vi "_sendCommand.vi"(8 "FBLR":dbl[](array[numeric]), 11 "error in (no error)":errorcluster) -> (3 "error out":errorcluster)   [LabVIEW 2021, in "System.lvclass"]
uses:
  System.lvclass
  <vilib>/myRIO/Instrument Drivers/Onboard IO/AO/typedefs/AO Reference.ctl
  <vilib>/myRIO/Common/Instrument Driver Framework/Utilities/typedefs/myRIO Generic Hardware Reference.ctl
  <vilib>/myRIO/Common/Instrument Driver Framework/Utilities/typedefs/Hardware Version Enum.ctl
  <vilib>/myRIO/Common/Instrument Driver Framework/Utilities/typedefs/myRIO v1.0 Reference.ctl
  <vilib>/myRIO/Common/Instrument Driver Framework/Utilities/typedefs/Generic FPGA Reference.ctl
  <vilib>/myRIO/Common/Instrument Driver Framework/myRIO v1.0/AO/typedefs/AO Channels List.ctl
  <vilib>/myRIO/Common/Instrument Driver Framework/myRIO v1.0/AO/typedefs/AO Channels Enum.ctl
  <vilib>/myRIO/Common/Instrument Driver Framework/Utilities/typedefs/Analog Scaling Constants List.ctl
  <vilib>/myRIO/Common/Instrument Driver Framework/Utilities/typedefs/Analog Scaling Constants.ctl
  <vilib>/userDefined/High Color/nirio_resource_hc.ctl
  <vilib>/myRIO/Common/Instrument Driver Framework/Utilities/vis/Is FPGA Ref Available.vi
  <vilib>/myRIO/Common/Instrument Driver Framework/myRIO v1.0/AO/vis/myRIO v1.1 Open AO.vi
  <vilib>/myRIO/Instrument Drivers/Onboard IO/AO/vis/Write.vi
  <vilib>/myRIO/Common/Instrument Driver Framework/Utilities/vis/Validate Channels.vi
  <vilib>/myRIO/Common/Instrument Driver Framework/myRIO v1.0/AO/vis/myRIO v1.0 Reserve AO.vi
  <vilib>/myRIO/Common/Instrument Driver Framework/myRIO v1.0/AO/vis/myRIO v1.0 Build MUX Configuration AO.vi
  <vilib>/myRIO/Common/Instrument Driver Framework/myRIO v1.0/Resource Manager/vis/myRIO v1.0 Reserve Channel List.vi
  <vilib>/myRIO/Common/Instrument Driver Framework/myRIO v1.0/Resource Manager/vis/myRIO v1.0 Reserve Channel.vi
  <vilib>/myRIO/Common/Instrument Driver Framework/myRIO v1.0/Resource Manager/vis/myRIO v1.0 Unreserve Channel.vi
  <vilib>/myRIO/Common/Instrument Driver Framework/myRIO v1.0/Resource Manager/vis/myRIO v1.0 Build Mutex Name.vi
  <vilib>/Utility/VariantDataType/GetNumericInfo.vi
  <vilib>/Utility/error.llb/Error Cluster From Error Code.vi
  <vilib>/myRIO/Common/Instrument Driver Framework/myRIO v1.0/myRIO v1.1 Open.vi
  <vilib>/myRIO/Common/Instrument Driver Framework/myRIO v1.0/AO/vis/myRIO v1.0 Get Scaling Constants AO.vi
  <vilib>/myRIO/Common/Instrument Driver Framework/Utilities/vis/IO Manager.vi
  <vilib>/myRIO/Common/Instrument Driver Framework/Utilities/vis/Configuration Manager.vi
  <vilib>/myRIO/Common/Instrument Driver Framework/myRIO v1.0/myRIO v1.0 Close.vi
  <vilib>/myRIO/Common/Instrument Driver Framework/myRIO v1.0/AO/vis/myRIO v1.0 Write AO.vi
  <vilib>/myRIO/Express VI/Onboard IO/AO/AO Express VI.xnode
  <vilib>/myRIO/Instrument Drivers/Onboard IO/AO/vis/myRIO AO Open.xnode
  <vilib>/myRIO/Instrument Drivers/Onboard IO/AO/AO.lvlib
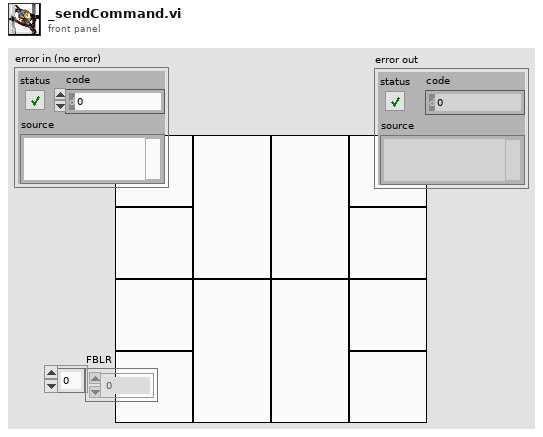
[diagram p1: front panel]
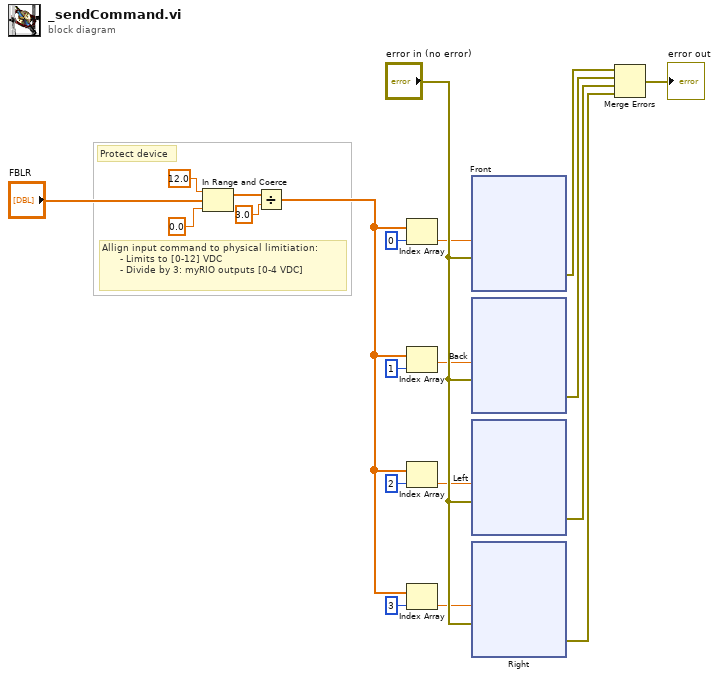
[diagram p0: block diagram]
diagram:
  # "Protect device"
  # "Allign input command to physical limitiation:\n      - Limits to [0-12] VDC\n      - Divide by 3: myRIO outputs [0-4 VDC]"
  n1 = In Range and Coerce(upper limit=12.0 ("y"), x="FBLR", lower limit=0.0 ("y")) -> (coerced(x)=w19:dbl[])  [unwired: 1 out]
  n2 = Divide(x=w19, y=3.0) -> (x/y=w18:dbl[])
  n3 = Index Array(array=w18, index=0) -> (element=w1:dbl)
  n4 = Index Array(array=w18, index=1) -> (element=w4:dbl)
  n5 = Index Array(array=w18, index=2) -> (element=w3:dbl)
  n6 = Index Array(array=w18, index=3) -> (element=w2:dbl)
  n7 = xnode "Front"("A/AO0 (Pin 2)"=w1, "error in (no error)"="error in (no error)") -> ("error out"=w10:errorcluster)
  n8 = xnode "Back"("A/AO1 (Pin 4)"=w4, "error in (no error)"="error in (no error)") -> ("error out"=w11:errorcluster)
  n9 = xnode "Left"("B/AO1 (Pin 4)"=w3, "error in (no error)"="error in (no error)") -> ("error out"=w12:errorcluster)
  n10 = xnode "Right"("B/AO0 (Pin 2)"=w2, "error in (no error)"="error in (no error)") -> ("error out"=w13:errorcluster)
  n11 = Merge Errors(w10, w11, w12, w13) -> (→"error out":errorcluster)
